vi "Main.vi"() -> ()   [LabVIEW 2018, in "TCP_Write.lvlib"]
doc: "This template is based off of the Queued Message Handler design pattern and the Queued Message Handler project template that ships with LabVIEW.\n\nThe main difference is that the queue is private to this module and communication between modules is performed via Broadcast and Request events.\n\nRequest events are wrapped in public API methods and are handled in the Event Handling Loop (EHL) of this VI. Any module can register for Broadcast events sent by this module. The EHL generates messages based on user interface actions.\n\nThe Message Handling Loop (MHL) processes messages generated by the EHL, or by other messages. The messages are string values, so new messages can be added easily to the Message Cases case structure in the MHL. Each message cluster can also provide an optional value for Message Data, which is a variant that can be converted to whatever message-specific data is required.\n_____\nBased on Delacor QMH Project Template 4.2.1.64."
uses:
  TCP_Write.lvlib
  <vilib>/Delacor/Delacor QMH/Libraries/Module Admin_class/Delacor_lib_QMH_Module Admin.lvclass
  Module Data--cluster.ctl
  Stop Argument--cluster.ctl
  <vilib>/Delacor/Delacor QMH/Libraries/Message Queue_class/Delacor_lib_QMH_Message Queue.lvclass/Delacor_lib_QMH_Message Queue.ctl
  <vilib>/Delacor/Delacor QMH/Libraries/Module Admin_class/Delacor_lib_QMH_Module Admin.lvclass/Delacor_lib_QMH_Module Admin.ctl
  Publish_Message Argument--cluster.ctl
  <vilib>/Utility/miscctls.llb/LVPointTypeDef.ctl
  <vilib>/Delacor/Delacor QMH/Libraries/Message Queue_class/Delacor_lib_QMH_Enqueue Message (Single).vi
  <vilib>/Delacor/Delacor QMH/Libraries/Module Admin_class/Delacor_lib_QMH_Get External Launch.vi
  <vilib>/Utility/error.llb/Error Cluster From Error Code.vi
  <vilib>/ErrorRing/Error Ring.xnode
  <vilib>/Delacor/Delacor QMH/Libraries/Message Queue_class/Delacor_lib_QMH_Message Queue.lvclass
panel:
  out "error out":errorcluster
  in  "Module Admin":refnum<class "Delacor_lib_QMH_Module Admin.lvclass">
  out "Status":string
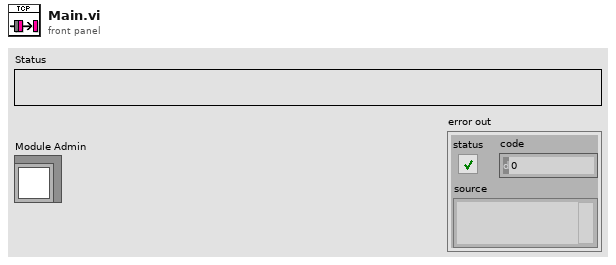
[diagram p1: front panel]
types:
  T1 = typedef "TCP_Write.lvlib/Request Events--cluster.ctl" = cluster{"Stop Module":refnum<user-event>, "Show Panel":refnum<user-event>, "Hide Panel":refnum<user-event>, "Get Module Execution Status":refnum<user-event>, "Show Diagram":refnum<user-event>, "Publish_Message":refnum<user-event>}
  T2 = typedef "TCP_Write.lvlib/Module Data--cluster.ctl" = cluster{"Status":string, "connection ID":refnum<k5>}
  T3 = enum32{"invalid lock state", "Not Locked", "Locked (No Password)", "Password-protected"}
  T4 = typedef "TCP_Write.lvlib/Stop Argument--cluster.ctl" = cluster{"Origin":string, "Exit via Stop Module Req?":bool, "Wait for Module to stop?":bool}
  T5 = typedef "TCP_Write.lvlib/Publish_Message Argument--cluster.ctl" = cluster{"Publish_Message":string}
  T6 = typedef "LVPointTypeDef.ctl" = cluster{"Horizontal":i16, "Vertical":i16}
  T7 = enum32{"Invalid", "Standard", "Closed", "Hidden", "Minimized", "Maximized"}
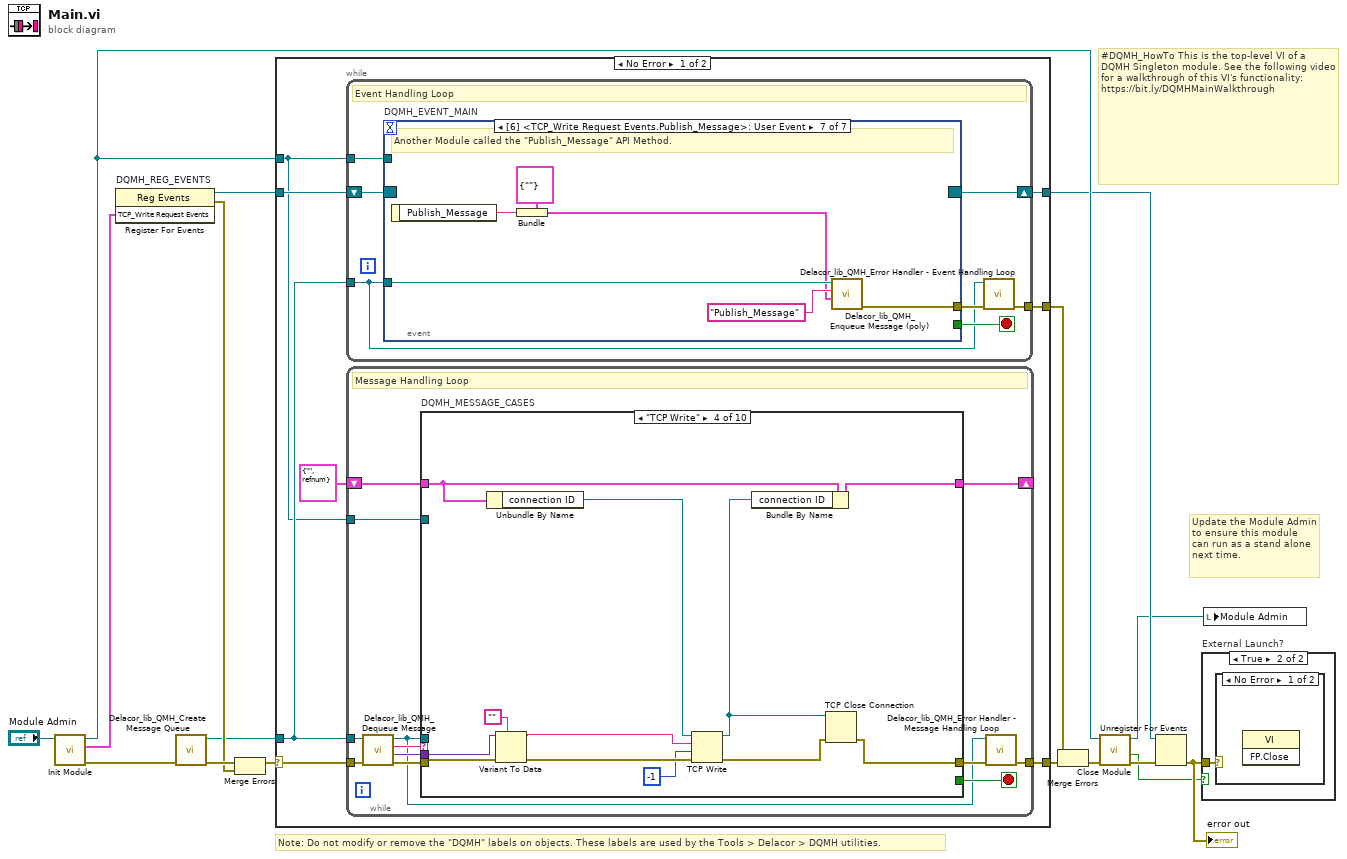
[diagram p0: block diagram]
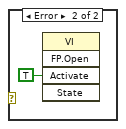
[diagram p3: hidden frame]
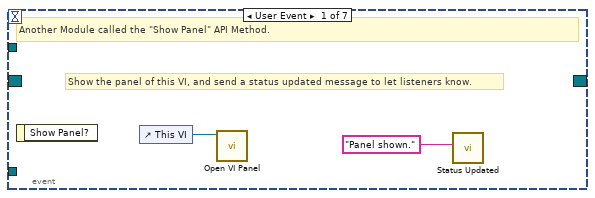
[diagram p4: hidden frame]
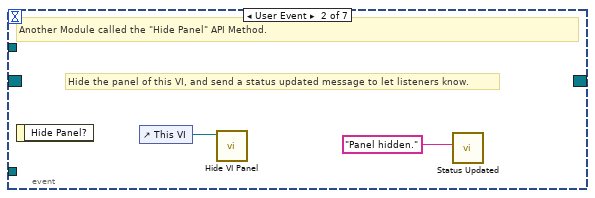
[diagram p5: hidden frame]
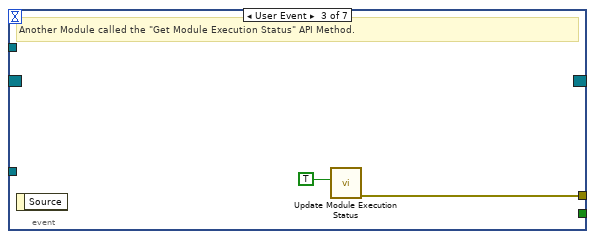
[diagram p6: hidden frame]
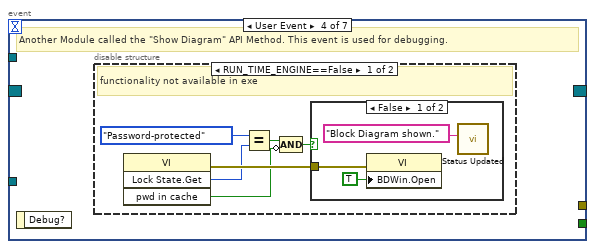
[diagram p7: hidden frame]
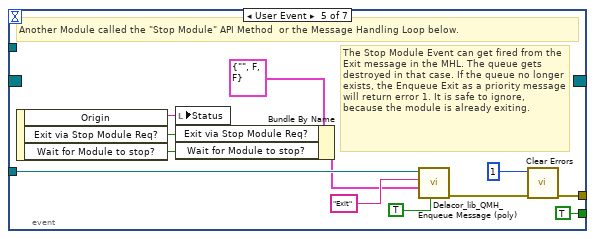
[diagram p10: hidden frame]
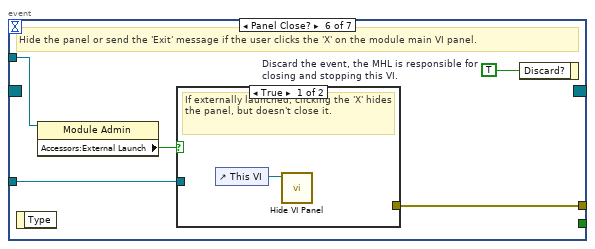
[diagram p11: hidden frame]
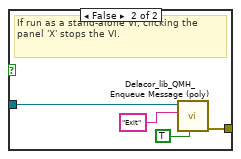
[diagram p12: hidden frame]
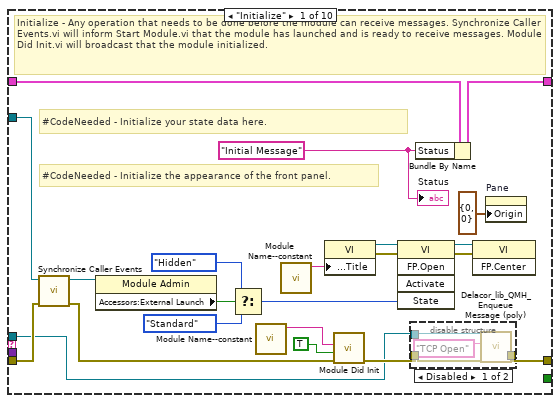
[diagram p13: hidden frame]
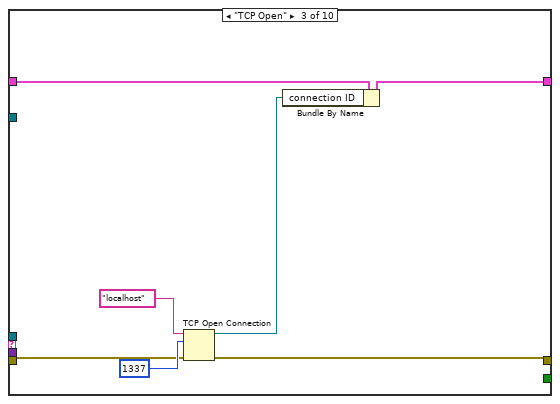
[diagram p16: hidden frame]
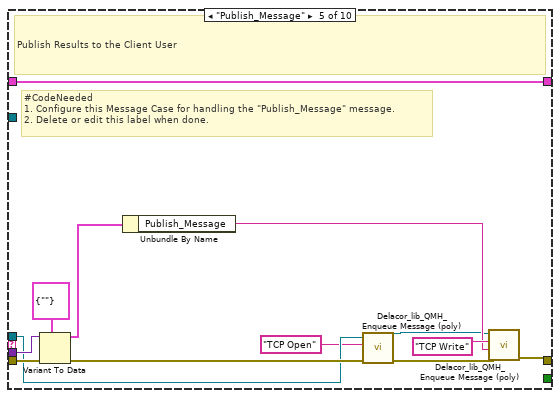
[diagram p17: hidden frame]
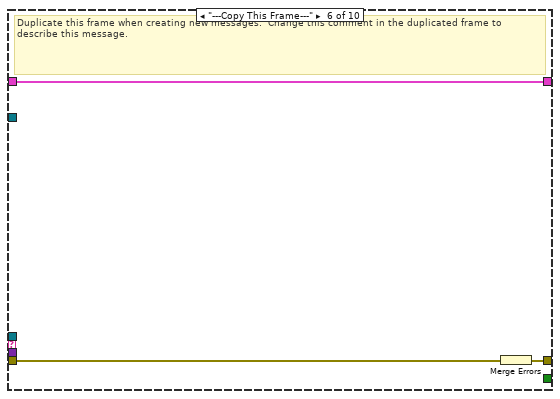
[diagram p18: hidden frame]
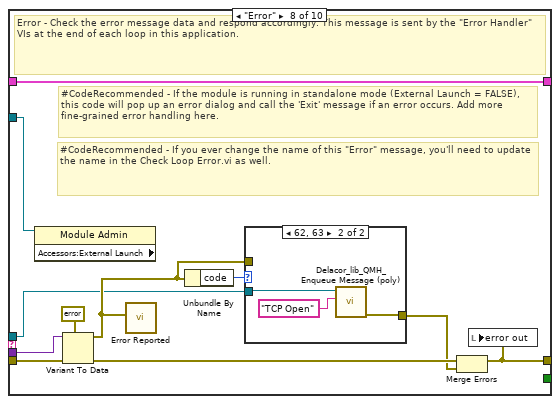
[diagram p20: hidden frame]
diagram:
  # "#DQMH_HowTo This is the top-level VI of a DQMH Singleton module. See the following video for a walkthrough of this VI's functionality: https://bit.ly/DQMHMainWalkthrough"
  # "Note: Do not modify or remove the \"DQMH\" labels on objects. These labels are used by the Tools > Delacor > DQMH utilities."
  # "Update the Module Admin to ensure this module can run as a stand alone next time."
  n1 = call "Init Module.vi"("Singleton Module Admin in"="Module Admin") -> ("error out"=w16:errorcluster, "TCP_Write Request Events"=w5:T1, "Singleton Module Admin out"=w8:refnum<class "Delacor_lib_QMH_Module Admin.lvclass">)  [unwired: 8 in]
  n2 = register-events "DQMH_REG_EVENTS"(w5) -> (reference out=w6:refnum<event-registration>, error out=w9:errorcluster)  [unwired: 2 in]
  n3 = call <vilib>:"Delacor_lib_QMH_Create Message Queue.vi"("error in (no error)"=w16) -> ("error out"=w11:errorcluster, "Message Queue"=w4:refnum<class "Delacor_lib_QMH_Message Queue.lvclass">)  [unwired: 9 in]
  n4 = Merge Errors(w11, w9) -> (w10:errorcluster)
  n5 = case shown="No Error" w10 {
    selector: w10 -> [w23 w210]
    tunnel: [w25 w210] -> w17
    tunnel: [w22 w207] -> w7
    tunnel: w6 -> [w20 w207]
    tunnel: w4 -> [w19 _]
    tunnel: [w24 _] -> w14
    tunnel: w8 -> [w18 w203]
    frame No Error {
      n6 = while {
        tunnel: w19 -> [w26]
        shift-right: [w29] -> w22
        shift-left: w20 -> [w30]
        tunnel: [w31] -> w24
        tunnel: w18 -> [w27]
        stop <- w28 stop-if-true
        # "Event Handling Loop"
        n7 = event "DQMH_EVENT_MAIN" shown="[6] <TCP_Write Request Events.Publish_Message>: User Event" {
          selector: w30 -> [_ _ _ _ _ _ _]
          dyn-events: [_ _ _ _ _ _ _] -> w29
          timeout: _ -> [_ _ _ _ _ _ _]
          tunnel: [_ _ _ _ TRUE ("Discard?") _ _] -> w28
          tunnel: w26 -> [_ _ _ _ w55 w62 w75]
          tunnel: [_ _ w38 _ w58 w64 w70] -> w32
          tunnel: w27 -> [_ _ _ _ _ w61 _]
          event User Event {
            # "Show the panel of this VI, and send a status updated message to let listeners know."
            # "Another Module called the \"Show Panel\" API Method."
            n8 = event-data() -> ()  [unwired: 1 in, 1 out]
            n9 = control-ref of="This VI"() -> (w34:refnum<vi>)
            n10 = call "Open VI Panel.vi"("VI"=w34) -> ()  [unwired: 10 in, 1 out]
            n11 = call "Status Updated.vi"("Status"="Panel shown." ("format string")) -> ()  [unwired: 10 in, 1 out]
          }
          event User Event {
            # "Hide the panel of this VI, and send a status updated message to let listeners know."
            # "Another Module called the \"Hide Panel\" API Method."
            n12 = event-data() -> ()  [unwired: 1 in, 1 out]
            n13 = control-ref of="This VI"() -> (w36:refnum<vi>)
            n14 = call "Hide VI Panel.vi"("VI"=w36) -> ()  [unwired: 10 in, 1 out]
            n15 = call "Status Updated.vi"("Status"="Panel hidden." ("format string")) -> ()  [unwired: 10 in, 1 out]
          }
          event User Event {
            # "Another Module called the \"Get Module Execution Status\" API Method."
            n16 = event-data() -> ()  [unwired: 1 in, 1 out]
            n17 = call "Update Module Execution Status.vi"("Running?"=TRUE) -> ("error out"=w38:errorcluster)  [unwired: 10 in]
          }
          event User Event {
            # "Another Module called the \"Show Diagram\" API Method. This event is used for debugging."
            n18 = event-data() -> ()  [unwired: 1 in, 1 out]
            n19 = disable-structure shown="RUN_TIME_ENGINE==False" {
              frame condition #0 (active) {
                # "functionality not available in exe"
                n20 = invoke class="VI" method="Lock State.Get"() -> (error out=w44:errorcluster, "Get Lock State"=w43:T3, "pwd in cache"=w40:bool)  [unwired: 4 in, 1 out]
                n21 = Equal?(x=T3."Password-protected", y=w43) -> (x = y?=w41:bool)
                n22 = Compound Arithmetic op=AND(w41, invert w40) -> (w39:bool)
                n23 = case shown="False" w39 {
                  tunnel: w44 -> [w47 _]
                  frame False {
                    n24 = property class="VI"(error in=w47, "BDWin.Open"=TRUE ("Block Diagram Window:Open")) -> ()  [unwired: 1 in, 2 out]
                    n25 = call "Status Updated.vi"("Status"="Block Diagram shown." ("format string")) -> ()  [unwired: 10 in, 1 out]
                  }
                  frame True {
                    # "Password-protected VI, and the password is not in the cache. Do not show the diagram."
                  }
                }
              }
              frame condition #1 {
              }
            }
          }
          event User Event {
            # "The Stop Module Event can get fired from the Exit message in the MHL. The queue gets destroyed in that case. If the queue no longer exists, the Enqueue Exit as a priority message will return error 1. It is safe to ignore, because the module is already exiting."
            # "Another Module called the \"Stop Module\" API Method  or the Message Handling Loop below."
            n26 = event-data() -> ("Origin"=w54:string, "Exit via Stop Module Req?"=w50:bool, "Wait for Module to stop?"=w49:bool)  [unwired: 1 in]
            n27 = local write "Status"(w54) -> ()
            n28 = Bundle By Name(cluster=T4 {"Origin"="", "Exit via Stop Module Req?"=FALSE, "Wait for Module to stop?"=FALSE} ("Stop Argument"), "Exit via Stop Module Req?"=w50, "Wait for Module to stop?"=w49) -> (w48:T4)
            n29 = call-poly <vilib>:"Delacor_lib_QMH_Enqueue Message (poly).vi"("Priority Message? (F)"=TRUE, "Message Data"=w48, "Message"="Exit", "Message Queue in"=w55) -> ("error out"=w59:errorcluster)  [unwired: 6 in, 1 out]
            n30 = call <vilib>:"Clear Errors.vi"("error in (no error)"=w59, "specific error code to clear (0: all)"=1) -> ("error out"=w58:errorcluster)  [unwired: 4 in, 1 out]
          }
          event Panel Close? {
            w63 = TRUE  # Discard the event, the MHL is responsible for closing and stopping this VI.
            # "Hide the panel or send the 'Exit' message if the user clicks the 'X' on the module main VI panel."
            n31 = event-data() -> ()  [unwired: 1 in, 1 out]
            n32 = property class="Module Admin"(reference=w61) -> ("Accessors:External Launch"=w60:bool)  [unwired: 1 in, 2 out]
            n33 = case shown="True" w60 {
              tunnel: w62 -> [_ w68]
              tunnel: [_ w69] -> w64
              frame True {
                # "If externally launched, clicking the 'X' hides the panel, but doesn't close it."
                n34 = control-ref of="This VI"() -> (w65:refnum<vi>)
                n35 = call "Hide VI Panel.vi"("VI"=w65) -> ()  [unwired: 10 in, 1 out]
              }
              frame False {
                # "If run as a stand-alone VI, clicking the panel 'X' stops the VI."
                n36 = call-poly <vilib>:"Delacor_lib_QMH_Enqueue Message (poly).vi"("Priority Message? (F)"=TRUE, "Message"="Exit", "Message Queue in"=w68) -> ("error out"=w69:errorcluster)  [unwired: 7 in, 1 out]
              }
            }
            n37 = event-data("Discard?"=w63) -> ()  [unwired: 1 in, 1 out]
          }
          event User Event {
            # "Another Module called the \"Publish_Message\" API Method."
            n38 = event-data() -> ("Publish_Message"=w71:string)  [unwired: 1 in]
            n39 = Bundle(cluster=T5 {"Publish_Message"=""} ("Publish_Message Argument"), "Publish_Message"=w71) -> (w72:T5)
            n40 = call-poly <vilib>:"Delacor_lib_QMH_Enqueue Message (poly).vi"("Message Data"=w72, "Message"="Publish_Message", "Message Queue in"=w75) -> ("error out"=w70:errorcluster)  [unwired: 7 in, 1 out]
          }
        }
        n41 = call-dynamic "Delacor_lib_QMH_Error Handler - Event Handling Loop.vi"("error in (no error)"=w32, "Message Queue in"=w26) -> ("dup error in"=w31:errorcluster)  [unwired: 8 in, 1 out]
      }
      n42 = while {
        tunnel: w19 -> [w78]
        shift-right: [w82] -> _
        shift-left: T2 {"Status"="", "connection ID"=refnum} ("Data Cluster") -> [w83]
        tunnel: w23 -> [w86]
        tunnel: [w84] -> w25
        tunnel: w18 -> [w76]
        stop <- w81 stop-if-true
        # "Message Handling Loop"
        n43 = call-dynamic "Delacor_lib_QMH_Dequeue Message.vi"("error in (no error)"=w86, "Message Queue in"=w78) -> ("error out"=w85:errorcluster, "Message Data"=w79:variant, "Message"=w80:string, "Message Queue out"=w77:refnum<class "Delacor_lib_QMH_Message Queue.lvclass">)  [unwired: 6 in]
        n44 = case "DQMH_MESSAGE_CASES" shown="\"TCP Write\"" w80 {
          selector: w80 -> [_ _ _ _ _ _ _ _ _ w190]
          tunnel: w77 -> [w88 _ _ _ w141 _ _ w155 w182 _]
          tunnel: w85 -> [w107 w115 w120 w134 w147 w150 w152 w162 w188 w192]
          tunnel: [w89 w115 w116 w123 w137 w149 w152 w158 w185 w193] -> w87
          tunnel: w83 -> [w97 w114 w122 w133 w146 w148 w151 w157 w173 w191]
          tunnel: [w96 w114 w118 w131 w146 w148 w151 w157 w173 w191] -> w82
          tunnel: [_ _ _ _ _ _ _ _ w181 _] -> w81
          tunnel: w79 -> [_ _ _ w129 w145 _ _ w156 w180 _]
          tunnel: w76 -> [w98 _ _ _ _ _ _ w154 w175 _]
          frame "Initialize" {
            w91 = "Initial Message" ("Initial Message")
            # "#CodeNeeded - Initialize the appearance of the front panel."
            # "#CodeNeeded - Initialize your state data here."
            # "Initialize - Any operation that needs to be done before the module can receive messages. Synchronize Caller Events.vi will inform Start Module.vi that the module has launched and is ready to receive messages. Module Did Init.vi will broadcast that the module initialized."
            n45 = call "Synchronize Caller Events.vi"("error in (no error)"=w107, "Singleton Module Admin in"=w98) -> ("error out"=w106:errorcluster, "Singleton Module Admin out"=w93:refnum<class "Delacor_lib_QMH_Module Admin.lvclass">)  [unwired: 8 in]
            n46 = property class="Module Admin"(reference=w93) -> ("Accessors:External Launch"=w102:bool)  [unwired: 1 in, 2 out]
            n47 = Select(t=T7."Hidden" ("State"), s=w102, f=T7."Standard" ("State")) -> (s? t:f=w99:T7)
            n48 = call "Module Name--constant.vi"() -> ("Module Name"=w94:string)  [unwired: 11 in]
            n49 = call "Module Name--constant.vi"() -> ("Module Name"=w105:string)  [unwired: 11 in]
            n50 = property class="VI"("Front Panel.Title"=w105) -> (reference out=w104:refnum<vi>, error out=w109:errorcluster)  [unwired: 2 in]
            n51 = call "Module Did Init.vi"("error in (no error)"=w106, "Initialized?"=TRUE, "Origin"=w94) -> ("error out"=w90:errorcluster)  [unwired: 8 in]
            n52 = invoke class="VI" method="FP.Open"(reference=w104, error in=w109, "State"=w99) -> (reference out=w103:refnum<vi>, error out=w108:errorcluster)  [unwired: 2 in, 3 out]
            n53 = disable-structure shown="Disabled" {
              disable-tunnel: w90 -> [w113 _]
              disable-tunnel: [w112 _] -> w89
              disable-tunnel: w88 -> [w111 _]
              frame Disabled {
                n54 = call-poly <vilib>:"Delacor_lib_QMH_Enqueue Message (poly).vi"("error in (no error)"=w113, "Message"="TCP Open", "Message Queue in"=w111) -> ("error out"=w112:errorcluster)  [unwired: 7 in, 1 out]
              }
              frame Enabled {
              }
            }
            n55 = Bundle By Name(cluster=w97, "Status"=w91) -> (w96:T2)
            n56 = invoke class="VI" method="FP.Center"(reference=w103, error in=w108) -> ()  [unwired: 1 in, 3 out]
            n57 = property on="Pane" class="Pane"("Origin"=T6 {"Horizontal"=0, "Vertical"=0}) -> ()  [unwired: 2 in, 2 out]
            "Status" <- w91
          }
          frame "--- Module Specific ---" {
            # "Separator -- The following cases handle messages specific to this Module."
          }
          frame "TCP Open" {
            n58 = TCP Open Connection(address="localhost", remote port or service name=u16 1337, error in (no error)=w120) -> (connection ID=w117:refnum<k5>, error out=w116:errorcluster)  [unwired: 2 in]
            n59 = Bundle By Name(cluster=w122, "connection ID"=w117) -> (w118:T2)
          }
          frame "TCP Write" {
            n60 = Unbundle By Name(w133) -> ("connection ID"=w132:refnum<k5>)
            n61 = Variant To Data(error in=w134, type="", Variant=w129) -> (data=w126:string, error out=w130:errorcluster)
            n62 = TCP Write(connection ID=w132, data in=w126, error in (no error)=w130, 9:-1 ("timeout ms (25000)")) -> (connection ID out=w125:refnum<k5>, error out=w124:errorcluster)  [unwired: 1 out]
            n63 = Bundle By Name(cluster=w133, "connection ID"=w125) -> (w131:T2)
            n64 = TCP Close Connection(connection ID=w125, error in (no error)=w124) -> (error out=w123:errorcluster)  [unwired: 1 in, 1 out]
          }
          frame "Publish_Message" {
            # "#CodeNeeded\n1. Configure this Message Case for handling the \"Publish_Message\" message.\n2. Delete or edit this label when done."
            # "Publish Results to the Client User"
            n65 = Variant To Data(error in=w147, type=T5 {"Publish_Message"=""} ("Publish_Message Argument"), Variant=w145) -> (data=w143:T5, error out=w142:errorcluster)
            n66 = Unbundle By Name(w143) -> ("Publish_Message"=w136:string)
            n67 = call-poly <vilib>:"Delacor_lib_QMH_Enqueue Message (poly).vi"("error in (no error)"=w142, "Message"="TCP Open", "Message Queue in"=w141) -> ("error out"=w138:errorcluster, "Message Queue out"=w135:refnum<class "Delacor_lib_QMH_Message Queue.lvclass">)  [unwired: 7 in]
            n68 = call-poly <vilib>:"Delacor_lib_QMH_Enqueue Message (poly).vi"("error in (no error)"=w138, "Message Data"=w136, "Message"="TCP Write", "Message Queue in"=w135) -> ("error out"=w137:errorcluster)  [unwired: 6 in, 1 out]
          }
          frame "---Copy This Frame---" {
            # "Duplicate this frame when creating new messages.  Change this comment in the duplicated frame to describe this message."
            n69 = Merge Errors(w150) -> (w149:errorcluster)
          }
          frame "--- Exit and Error Handling---" {
            # "Separator - The following cases handle errors and exit messages."
          }
          frame "Error" {
            # "#CodeRecommended - If you ever change the name of this \"Error\" message, you'll need to update the name in the Check Loop Error.vi as well."
            # "#CodeRecommended - If the module is running in standalone mode (External Launch = FALSE), this code will pop up an error dialog and call the 'Exit' message if an error occurs. Add more fine-grained error handling here."
            # "Error - Check the error message data and respond accordingly. This message is sent by the \"Error Handler\" VIs at the end of each loop in this application."
            n70 = property class="Module Admin" props=["Accessors:External Launch"](reference=w154) -> ()  [unwired: 1 in, 3 out]
            n71 = Variant To Data(error in=w162, type=errorcluster {"status"=FALSE, "code"=0, "source"=""} ("error constant"), Variant=w156) -> (data=w163:errorcluster, error out=w160:errorcluster)
            n72 = call "Error Reported.vi"("Error"=w163) -> ()  [unwired: 10 in, 1 out]
            n73 = Unbundle By Name(w163) -> ("code"=w153:i32)
            n74 = case shown="62, 63" w153 {
              tunnel: [w168 w169] -> w159
              tunnel: w155 -> [w167 w170]
              tunnel: w163 -> [w164 _]
              frame Default {
                n75 = call <vilib>:"Simple Error Handler.vi"("error in (no error)"=w164) -> ()  [unwired: 4 in, 5 out]
                n76 = call-poly <vilib>:"Delacor_lib_QMH_Enqueue Message (poly).vi"("Priority Message? (F)"=TRUE, "Message"="Exit", "Message Queue in"=w167) -> ("error out"=w168:errorcluster)  [unwired: 7 in, 1 out]
              }
              frame 62, 63 {
                n77 = call-poly <vilib>:"Delacor_lib_QMH_Enqueue Message (poly).vi"("Message"="TCP Open", "Message Queue in"=w170) -> ("error out"=w169:errorcluster)  [unwired: 8 in, 1 out]
              }
            }
            n78 = Merge Errors(w160, w159) -> (w158:errorcluster)
            n79 = local write "error out"(w158) -> ()
          }
          frame "Exit" {
            w179 = 91  # 91: not all Exit messages will have an argument
            w181 = TRUE  # Stop the VI
            # "Release the message queue reference"
            # "#CodeNeeded - Add any required cleanup code here"
            # "Exit - Exit the application."
            n80 = Unbundle By Name(w173) -> ("connection ID"=w172:refnum<k5>)
            n81 = Variant To Data(error in=w188, type=T4 {"Origin"="", "Exit via Stop Module Req?"=FALSE, "Wait for Module to stop?"=FALSE} ("Stop Argument"), Variant=w180) -> (data=w177:T4, error out=w184:errorcluster)
            n82 = call <vilib>:"Clear Errors.vi"("error in (no error)"=w184, "specific error code to clear (0: all)"=w179) -> ("error out"=w187:errorcluster)  [unwired: 4 in, 1 out]
            n83 = TCP Close Connection(connection ID=w172, error in (no error)=w187) -> (error out=w174:errorcluster)  [unwired: 1 in, 1 out]
            n84 = control-ref of="This VI"() -> (w176:refnum<vi>)
            n85 = call-dynamic "Delacor_lib_QMH_Release Message Queue.vi"("error in (no error)"=w174, "Message Queue"=w182) -> ("error out"=w186:errorcluster)  [unwired: 9 in]
            n86 = call "Handle Exit.vi"("Stop Argument"=w177, "Admin in"=w175, "VI reference"=w176) -> ("error out"=w183:errorcluster)  [unwired: 7 in, 1 out]
            n87 = Merge Errors(w186, w183) -> (w185:errorcluster)
          }
          frame Default {
            # "'Default' case only runs if there is a message that isn't defined in any of the other cases.  Output a programming error."
            n88 = call "Module Name--constant.vi"() -> ("Module Name"=w189:string)  [unwired: 11 in]
            n89 = xnode "Error Ring"("parameter 0"=w190, "parameter 1"=w189) -> ("error out"=w194:errorcluster)
            n90 = Merge Errors(w192, w194) -> (w193:errorcluster)
          }
        }
        n91 = call-dynamic "Delacor_lib_QMH_Error Handler - Message Handling Loop.vi"("error in (no error)"=w87, "Message Queue in"=w77) -> ("dup error in"=w84:errorcluster)  [unwired: 8 in, 1 out]
      }
    }
    frame Error {
      # "Synchronize Caller Events.vi will inform Start Module.vi that the module has launched and will let the code calling Start Module.vi register for broadcasts and would permit the caller receive the broadcast that an error occurred at launch time."
      n92 = call "Synchronize Caller Events.vi"("Singleton Module Admin in"=w203) -> ("error out"=w208:errorcluster)  [unwired: 9 in, 1 out]
      n93 = call "Module Name--constant.vi"() -> ("Module Name"=w206:string)  [unwired: 11 in]
      n94 = Format Into String(format string="An error occurred during initialization. %s is no longer running.", w206) -> (resulting string=w204:string)  [unwired: 2 in, 1 out]
      n95 = Merge Errors(w210, w208) -> (w209:errorcluster)
      n96 = call "Error Reported.vi"("Additional Information"=w204, "Error"=w209) -> ()  [unwired: 9 in, 1 out]
    }
  }
  n97 = Merge Errors(w14, w17) -> (w13:errorcluster)
  n98 = call "Close Module.vi"("error in (no error)"=w13, "Module Admin in"=w8) -> ("error out"=w15:errorcluster, "External Launch"=w1:bool, "Module Admin out"=w2:refnum<class "Delacor_lib_QMH_Module Admin.lvclass">)  [unwired: 7 in]
  n99 = Unregister For Events(event registration refnum=w7, error in=w15) -> (error out=w12:errorcluster)
  "error out" <- w12
  n100 = case "External Launch?" shown="True" w1 {
    tunnel: w12 -> [_ w211]
    frame False {
    }
    frame True {
      n101 = case shown="No Error" w211 {
        frame No Error {
          n102 = invoke class="VI" method="FP.Close"() -> ()  [unwired: 3 in, 3 out]
        }
        frame Error {
          n103 = invoke class="VI" method="FP.Open"("Activate"=TRUE ("Activate?")) -> ()  [unwired: 4 in, 5 out]
        }
      }
    }
  }
  n104 = local write "Module Admin"(w2) -> ()
